vi "inteference V1.vi"(7 "number of points":i32, 8 "complex region":T1={"max re"=5.161869466666667e-06, "min re"=5.176843333333334e-06, "max im"=-2.467216e-05, "min im"=-0.001573233, "delta re"=0.003211203, "delta im"=0.00165815, "center re"=0.0015485608400000002, "delta  z"=0.0015530530000000002+0.0i, "center im"=0.0, "center z"=0.0+0.0i, "d im"=0.0, "d re"=0.0, "d z"=0.0+0.0i}, 9 "bathtub":cdb[][](array[numeric]), 10 "point sources":cdb[](array[numeric]), 11 "wave packet":cdb[][](array[numeric])) -> (3 "bathtub out":cdb[][](array[numeric]))   [LabVIEW 2010]
uses:
  complex region.ctl
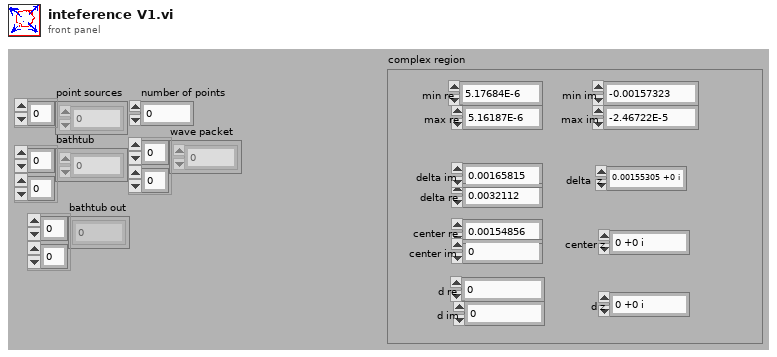
[diagram p1: front panel]
types:
  T1 = typedef "complex region.ctl" = cluster{"max re":dbl, "min re":dbl, "max im":dbl, "min im":dbl, "delta re":dbl, "delta im":dbl, "center re":dbl, "delta  z":cdb, "center im":dbl, "center z":cdb, "d im":dbl, "d re":dbl, "d z":cdb}
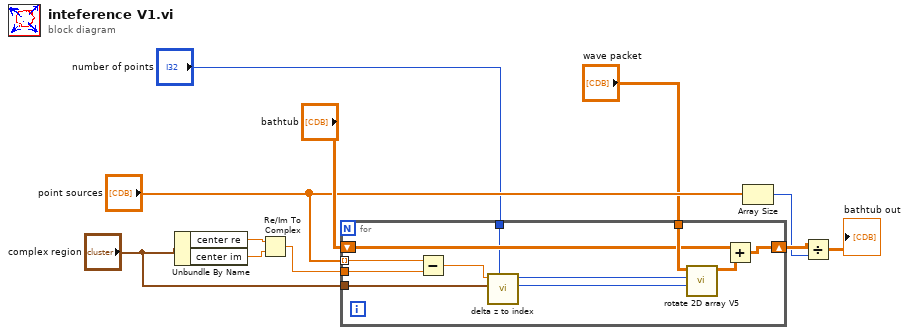
[diagram p0: block diagram]
diagram:
  n1 = Unbundle By Name("complex region") -> ("center re"=w11:dbl, "center im"=w10:dbl)
  n2 = Re/Im To Complex(1:w10, 2:w11) -> (0:w9:cdb)
  n3 = for {
    shift-right: [w19] -> w8
    shift-left: "bathtub" -> [w21]
    tunnel: "point sources" -> [w15] mode=indexing
    tunnel: "wave packet" -> [w22]
    tunnel: "complex region" -> [w18]
    tunnel: w9 -> [w14]
    tunnel: "number of points" -> [w12]
    n4 = Subtract(x=w15, y=w14) -> (x-y=w13:cdb)
    n5 = call "delta z to index.vi"("number of points"=w12, "complex region"=w18, "z"=w13) -> ("im index"=w16:i32, "re index"=w17:i32)  [unwired: 7 in]
    n6 = call "rotate 2D array V5.vi"("rotate y"=w16, "rotate x"=w17, "array in"=w22) -> ("array out"=w20:cdb[][])  [unwired: 8 in]
    n7 = Add(x=w21, y=w20) -> (x+y=w19:cdb[][])
  }
  n8 = Array Size(array="point sources") -> (size(s)=w7:i32)
  n9 = Divide(x=w8, y=w7) -> (x/y=→"bathtub out":cdb[][])
